vi "Reset Count.vi"   [LabVIEW 2015, in "Agilent 2000 3000 X-Series.lvlib"]
doc: "Resets frame counters."
uses:
  <instrlib>/Agilent 2000 3000 X-Series/Agilent 2000 3000 X-Series.lvlib
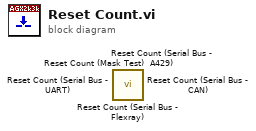
[diagram p0: block diagram]
diagram:
  n1 = call <instrlib>:"Reset Count (Serial Bus - Flexray).vi"() -> ()  [unwired: 10 in, 2 out]
  n2 = call <instrlib>:"Reset Count (Serial Bus - A429).vi"() -> ()  [unwired: 10 in, 2 out]
  n3 = call <instrlib>:"Reset Count (Serial Bus - UART).vi"() -> ()  [unwired: 10 in, 2 out]
  n4 = call <instrlib>:"Reset Count (Serial Bus - CAN).vi"() -> ()  [unwired: 10 in, 2 out]
  n5 = call <instrlib>:"Reset Count (Mask Test).vi"() -> ()  [unwired: 10 in, 2 out]
